vi "SVXMPL_Get Wav List.vi"(7 "name of the file":string, 8 "error in (no error)":errorcluster) -> (0 "error out":errorcluster, 1 "example data folder":path, 2 "Path":path[](array[path]), 3 "file names":string[](array[string]), 4 "index":i32, 5 "appended path":path)   [LabVIEW 2017]
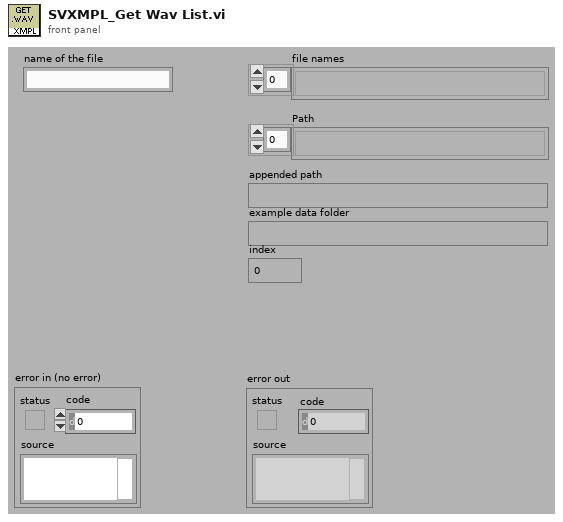
[diagram p1: front panel]
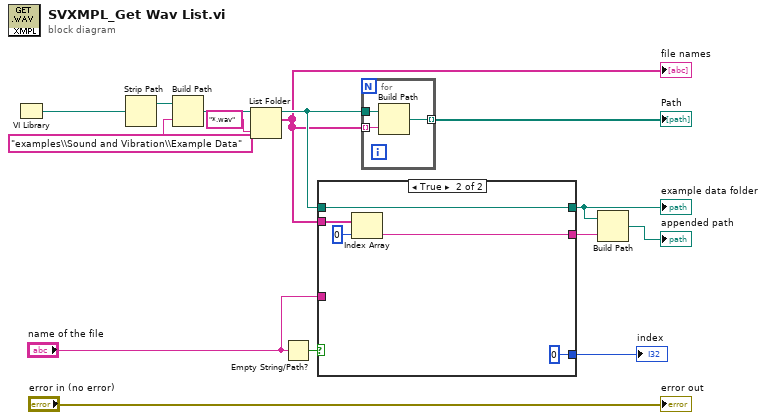
[diagram p0: block diagram]
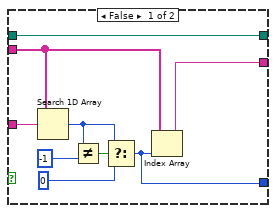
[diagram p2: hidden frame]
diagram:
  n1 = VI Library() -> (path=w12:path)
  n2 = Strip Path(path=w12) -> (stripped path=w13:path)  [unwired: 1 out]
  n3 = Build Path(base path=w13, name or relative path="examples\\Sound and Vibration\\Example Data") -> (appended path=w11:path)
  n4 = List Folder(path=w11, pattern="*.wav") -> (path out=w6:path, filenames=w5:string[])  [unwired: 2 in, 2 out]
  "file names" <- w5
  n5 = Empty String/Path?(string/path="name of the file") -> (empty?=w8:bool)
  n6 = case shown="True" w8 {
    tunnel: w5 -> [w20 w28]
    tunnel: "name of the file" -> [w24 _]
    tunnel: w6 -> [w23 w29]
    tunnel: [w23 w29] -> w3
    tunnel: [w17 w27] -> w4
    tunnel: [w16 0] -> w1
    frame False {
      n7 = Search 1D Array(1D array=w20, element=w24) -> (index of element=w18:i32)  [unwired: 1 in]
      n8 = Not Equal?(x=w18, y=-1) -> (x != y?=w21:bool)
      n9 = Select(t=w18, s=w21, f=0 ("Index")) -> (s? t:f=w16:i32)
      n10 = Index Array(array=w20, index=w16) -> (element=w17:string)
    }
    frame True {
      n11 = Index Array(array=w28, index=0 ("Index")) -> (element=w27:string)
    }
  }
  "example data folder" <- w3
  "index" <- w1
  n12 = for {
    tunnel: [w32] -> w9 mode=indexing
    tunnel: w6 -> [w31]
    tunnel: w5 -> [w30] mode=indexing
    n13 = Build Path(base path=w31, name or relative path=w30) -> (appended path=w32:path)
  }
  "Path" <- w9
  n14 = Build Path(base path=w3, name or relative path=w4) -> (appended path=→"appended path":path)
  "error out" <- "error in (no error)"
